vi "Update Map.vi"(9 "Action":T2, 10 "Direction":T1, 11 "Class":refnum<class "Hesitant Wolf.lvclass">) -> (3 "Class":refnum<class "Hesitant Wolf.lvclass">)   [LabVIEW 2015, in "Hesitant Wolf.lvclass"]
uses:
  Hesitant Wolf.lvclass
  Type Defs/Action Enum.ctl
  Type Defs/Direction Enum.ctl
  Hesitant Wolf.lvclass/Hesitant Wolf.ctl
  SubVIs/Read-Only Globals.vi
  Square/Square.lvclass
  Type Defs/SB Type Defs.lvlib
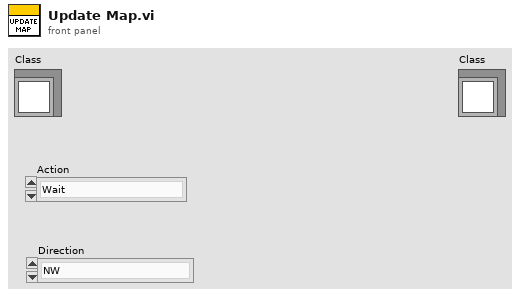
[diagram p1: front panel]
types:
  T1 = typedef "SB Type Defs.lvlib/Direction Enum.ctl" = enum16{"NW", "N", "NE", "E", "SE", "S", "SW", "W"}
  T2 = typedef "SB Type Defs.lvlib/Action Enum.ctl" = enum16{"Wait", "Move", "Attack", "Replicate"}
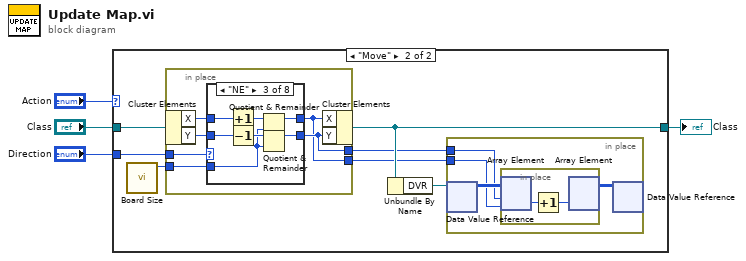
[diagram p0: block diagram]
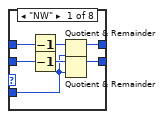
[diagram p3: hidden frame]
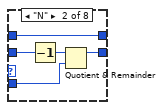
[diagram p4: hidden frame]
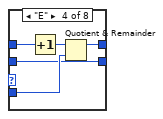
[diagram p5: hidden frame]
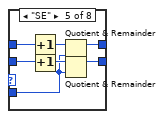
[diagram p6: hidden frame]
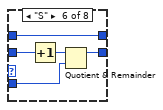
[diagram p7: hidden frame]
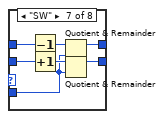
[diagram p8: hidden frame]
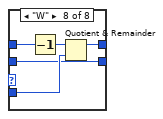
[diagram p9: hidden frame]
diagram:
  n1 = case shown="\"Move\"" "Action" {
    tunnel: "Class" -> [w5 w12]
    tunnel: [w5 w9] -> w2
    tunnel: "Direction" -> [_ w11]
    frame Default {
    }
    frame "Move" {
      n2 = call "Board Size.vi"() -> ("Board Size"=w10:i32)  [unwired: 11 in]
      n3 = in-place {
        in-place-border: w11 -> [w24]
        in-place-border: w10 -> [w21]
        in-place-border: [w20] -> w7
        in-place-border: [w19] -> w6
        n4 = in-place-cluster #1(w12) -> ("X"=w23:i32, "Y"=w22:i32)
        n5 = case shown="\"NE\"" w24 {
          tunnel: w23 -> [w30 w32 w42 w48 w54 w56 w66 w72]
          tunnel: w22 -> [w31 w36 w43 w44 w55 w60 w67 w68]
          tunnel: [w28 w34 w40 w44 w52 w58 w64 w68] -> w20
          tunnel: [w25 w32 w37 w45 w49 w56 w61 w69] -> w19
          tunnel: w21 -> [w26 w33 w38 w46 w50 w57 w62 w70]
          frame "NW" {
            n6 = Decrement(x=w30) -> (x-1=w27:i32)
            n7 = Decrement(x=w31) -> (x-1=w29:i32)
            n8 = Quotient & Remainder(x=w27, y=w26) -> (x-y*floor(x/y)=w25:i32)  [unwired: 1 out]
            n9 = Quotient & Remainder(x=w29, y=w26) -> (x-y*floor(x/y)=w28:i32)  [unwired: 1 out]
          }
          frame "N" {
            n10 = Decrement(x=w36) -> (x-1=w35:i32)
            n11 = Quotient & Remainder(x=w35, y=w33) -> (x-y*floor(x/y)=w34:i32)  [unwired: 1 out]
          }
          frame "NE" {
            n12 = Increment(x=w42) -> (x+1=w39:i32)
            n13 = Decrement(x=w43) -> (x-1=w41:i32)
            n14 = Quotient & Remainder(x=w39, y=w38) -> (x-y*floor(x/y)=w37:i32)  [unwired: 1 out]
            n15 = Quotient & Remainder(x=w41, y=w38) -> (x-y*floor(x/y)=w40:i32)  [unwired: 1 out]
          }
          frame "E" {
            n16 = Increment(x=w48) -> (x+1=w47:i32)
            n17 = Quotient & Remainder(x=w47, y=w46) -> (x-y*floor(x/y)=w45:i32)  [unwired: 1 out]
          }
          frame "SE" {
            n18 = Increment(x=w54) -> (x+1=w51:i32)
            n19 = Increment(x=w55) -> (x+1=w53:i32)
            n20 = Quotient & Remainder(x=w51, y=w50) -> (x-y*floor(x/y)=w49:i32)  [unwired: 1 out]
            n21 = Quotient & Remainder(x=w53, y=w50) -> (x-y*floor(x/y)=w52:i32)  [unwired: 1 out]
          }
          frame "S" {
            n22 = Increment(x=w60) -> (x+1=w59:i32)
            n23 = Quotient & Remainder(x=w59, y=w57) -> (x-y*floor(x/y)=w58:i32)  [unwired: 1 out]
          }
          frame "SW" {
            n24 = Decrement(x=w66) -> (x-1=w63:i32)
            n25 = Increment(x=w67) -> (x+1=w65:i32)
            n26 = Quotient & Remainder(x=w63, y=w62) -> (x-y*floor(x/y)=w61:i32)  [unwired: 1 out]
            n27 = Quotient & Remainder(x=w65, y=w62) -> (x-y*floor(x/y)=w64:i32)  [unwired: 1 out]
          }
          frame "W" {
            n28 = Decrement(x=w72) -> (x-1=w71:i32)
            n29 = Quotient & Remainder(x=w71, y=w70) -> (x-y*floor(x/y)=w69:i32)  [unwired: 1 out]
          }
        }
        n30 = in-place-cluster #1("X"=w19, "Y"=w20) -> (w9:refnum<class "Hesitant Wolf.lvclass">)
      }
      n31 = Unbundle By Name(w9) -> ("DVR"=w8:refnum<data-value>)
      n32 = in-place {
        in-place-border: w7 -> [w15]
        in-place-border: w6 -> [w14]
        n33 = in-place-dvr #2(w8) -> (w16:i32[][])  [unwired: 1 out]
        n34 = in-place {
          n35 = in-place-array #3(w16, w15, w14) -> (w18:i32)
          n36 = Increment(x=w18) -> (x+1=w17:i32)
          n37 = in-place-array #3(w17) -> (w13:i32[][])  [unwired: 2 out]
        }
        n38 = in-place-dvr #2(w13) -> ()  [unwired: 2 out]
      }
    }
  }
  "Class" <- w2
